vi "HMI-Reactor.vi"() -> ()   [LabVIEW 2018]
uses:
  <vilib>/Platform/TimedLoop/XDataNode/timing_clust.ctl
  <vilib>/Platform/TimedLoop/XDataNode/nitl_modes.ctl
  <vilib>/Platform/TimedLoop/XDataNode/wakeup.ctl
  <vilib>/Modbus/master/Create Master Instance (TCP).vi
  <vilib>/Modbus/master/Modbus Master.lvclass
  <vilib>/Platform/TimedLoop/XDataNode/XDataNode.xnode
  <vilib>/Platform/TimedLoop/XDataNode/XDNodeRunTimeDep.lvlib
panel:
  out "BPCS-10HIC100":dbl
  out "BPCS-10TIC100-SP":dbl
  out "BPCS-10TIC100-KD":dbl
  out "BPCS-10TIC100-KI":dbl
  out "BPCS-10TIC100-KP":dbl
  out "BPCS-10HIC200":dbl
  out "BPCS-10LIC200-SP":dbl
  out "BPCS-10LIC200-KD":dbl
  out "BPCS-10LIC200-KI":dbl
  out "BPCS-10LIC200-KP":dbl
  out "BPCS-10HIC300":dbl
  in  "cast type 3":dbl[](array[numeric])
  out "M2":bool
  out "M1":bool
  in  "type":u16[](array[numeric])
  in  "cast type 2":dbl[](array[numeric])
  out "F":dbl
  in  "cast type":dbl[](array[numeric])
  out "CA":dbl=456.3558684423593 format="%#_3g"
  out "CA0":dbl=2000.0 format="%#_3g"
  out "10SDV502":bool=TRUE
  out "?":dbl format="%#_3g"
  in  "10HIC300":dbl=50.0
  out "TJ":dbl=365.3749789937039 format="%#_3g"
  out "T":dbl=333.97788169438996 format="%#_3g"
  out "Reactor Temp":T1={"% Opening"=0.0, "SP"=0.0, "Reactor Temp"=333.97788169438996, "Temp"=333.97788169438996} {"Temp" format="%#_4g"; "Reactor Temp" scale=0.0..700.0; "SP" scale=0.0..700.0; "% Opening" scale=0.0..100.0}
  in  "10TIC100 Faceplate":T2={"PID Parameters"={"KP"=-1.0, "KI"=0.5, "KD"=0.0}, "M"=FALSE, "SP_VAL"=0.0, "% Open"=50.0}
  out "?":dbl format="%#_3g"
  out "10SDV501":bool=TRUE
  out "FJ":dbl=15.0 format="%#_3g"
  out "TJ0":dbl=300.0 format="%#_3g"
  out "10SDV500":bool=TRUE
  out "F0":dbl=1.0 format="%#_3g"
  out "T0":dbl=323.0 format="%#_3g"
  out "Reactor Level":T3={"% Opening"=0.0, "SP"=0.0, "Reactor Level"=54.508701366151044, "Level"=54.508701366151044} {"Level" format="%#_4g"; "Reactor Level" scale=0.0..100.0; "SP" scale=0.0..100.0; "% Opening" scale=0.0..100.0}
  out "?":dbl format="%#_3g"
  in  "10LIC200 Faceplate":T2={"PID Parameters"={"KP"=8.0, "KI"=0.4, "KD"=0.0}, "M"=FALSE, "SP_VAL"=0.0, "% Open"=50.0}
  out "10-R-100":dbl(slide)=54.508701366151044 scale=0.0..100.0 scale format="%#_4g"
  in  "stop":bool
  # "LIC = level controller"
  # "feed flow"
  # "Reactant inlet concentration"
  # "m3/min"
  # "10LV200"
  # "Mole/m3"
  # "%"
  # "K"
  # "%"
  # "K"
  # "TIC=Temperature controller"
  # "coolant flow"
  # "m3/min"
  # "10TV100"
  # "%"
  # "K"
  # "Mole/m3"
  # "%"
  # "K"
  # "coolant inlet temp"
  # "A"
  # "%"
  # "A"
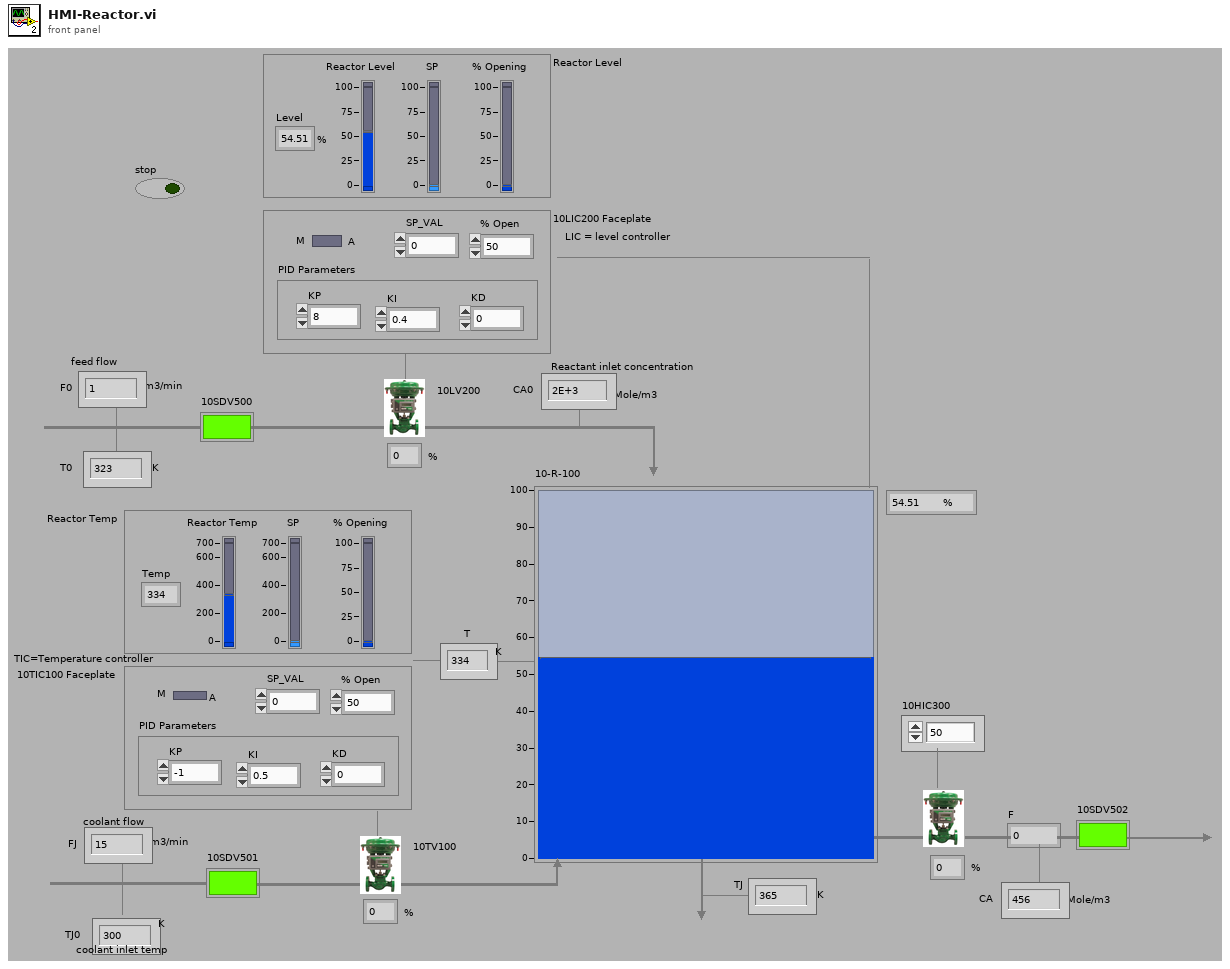
[diagram p1: front panel]
types:
  T1 = cluster{"% Opening":dbl, "SP":dbl, "Reactor Temp":dbl, "Temp":dbl}
  T2 = cluster{"PID Parameters":cluster{"KP":dbl, "KI":dbl, "KD":dbl}, "M":bool, "SP_VAL":dbl, "% Open":dbl}
  T3 = cluster{"% Opening":dbl, "SP":dbl, "Reactor Level":dbl, "Level":dbl}
  T4 = typedef "XDNodeRunTimeDep.lvlib/timing_clust.ctl" = cluster{"Expected End [f-1]":u64, "Actual End [f-1]":u64, "Finished Late? [f-1]":bool, "Expected End [i-1]":u64, "Actual End [i-1]":u64, "Finished Late? [i-1]":bool, "Expected Start [i]":u64, "Actual Start [i]":u64, "Expected Start [f]":u64, "Actual Start [f]":u64, "Source Name":string, "Structure Name":string, "Period":i64, "Deadline":i64, "Offset":i64, "Start":i64, "Priority":i32, "Timeout":i32, "Mode":T5, "Wakeup Reason":T6, "Error":errorcluster, "Source Type":string, "Secondary Source Type":string, "Global End Time":u64, "Global Start Time":u64, "Frame Duration":u64, "Iteration Duration":u64, "Assigned CPU":i32, "I/O Scan Engine Mode":u32}
  T5 = typedef "XDNodeRunTimeDep.lvlib/nitl_modes.ctl" = enum32{"No Change", "Process missed periods, maintain original phase", "Discard missed periods, maintain original phase", "Process missed periods, ignore original phase", "Discard missed periods, ignore original phase"}
  T6 = typedef "XDNodeRunTimeDep.lvlib/wakeup.ctl" = enum32{"Normal", "Aborted", "Asynchronous wakeup", "Timing source error", "Timed loop error", "Timeout"}
  T7 = cluster{"% Open":dbl, "SP_VAL":dbl, "Numeric":dbl, "Numeric":dbl}
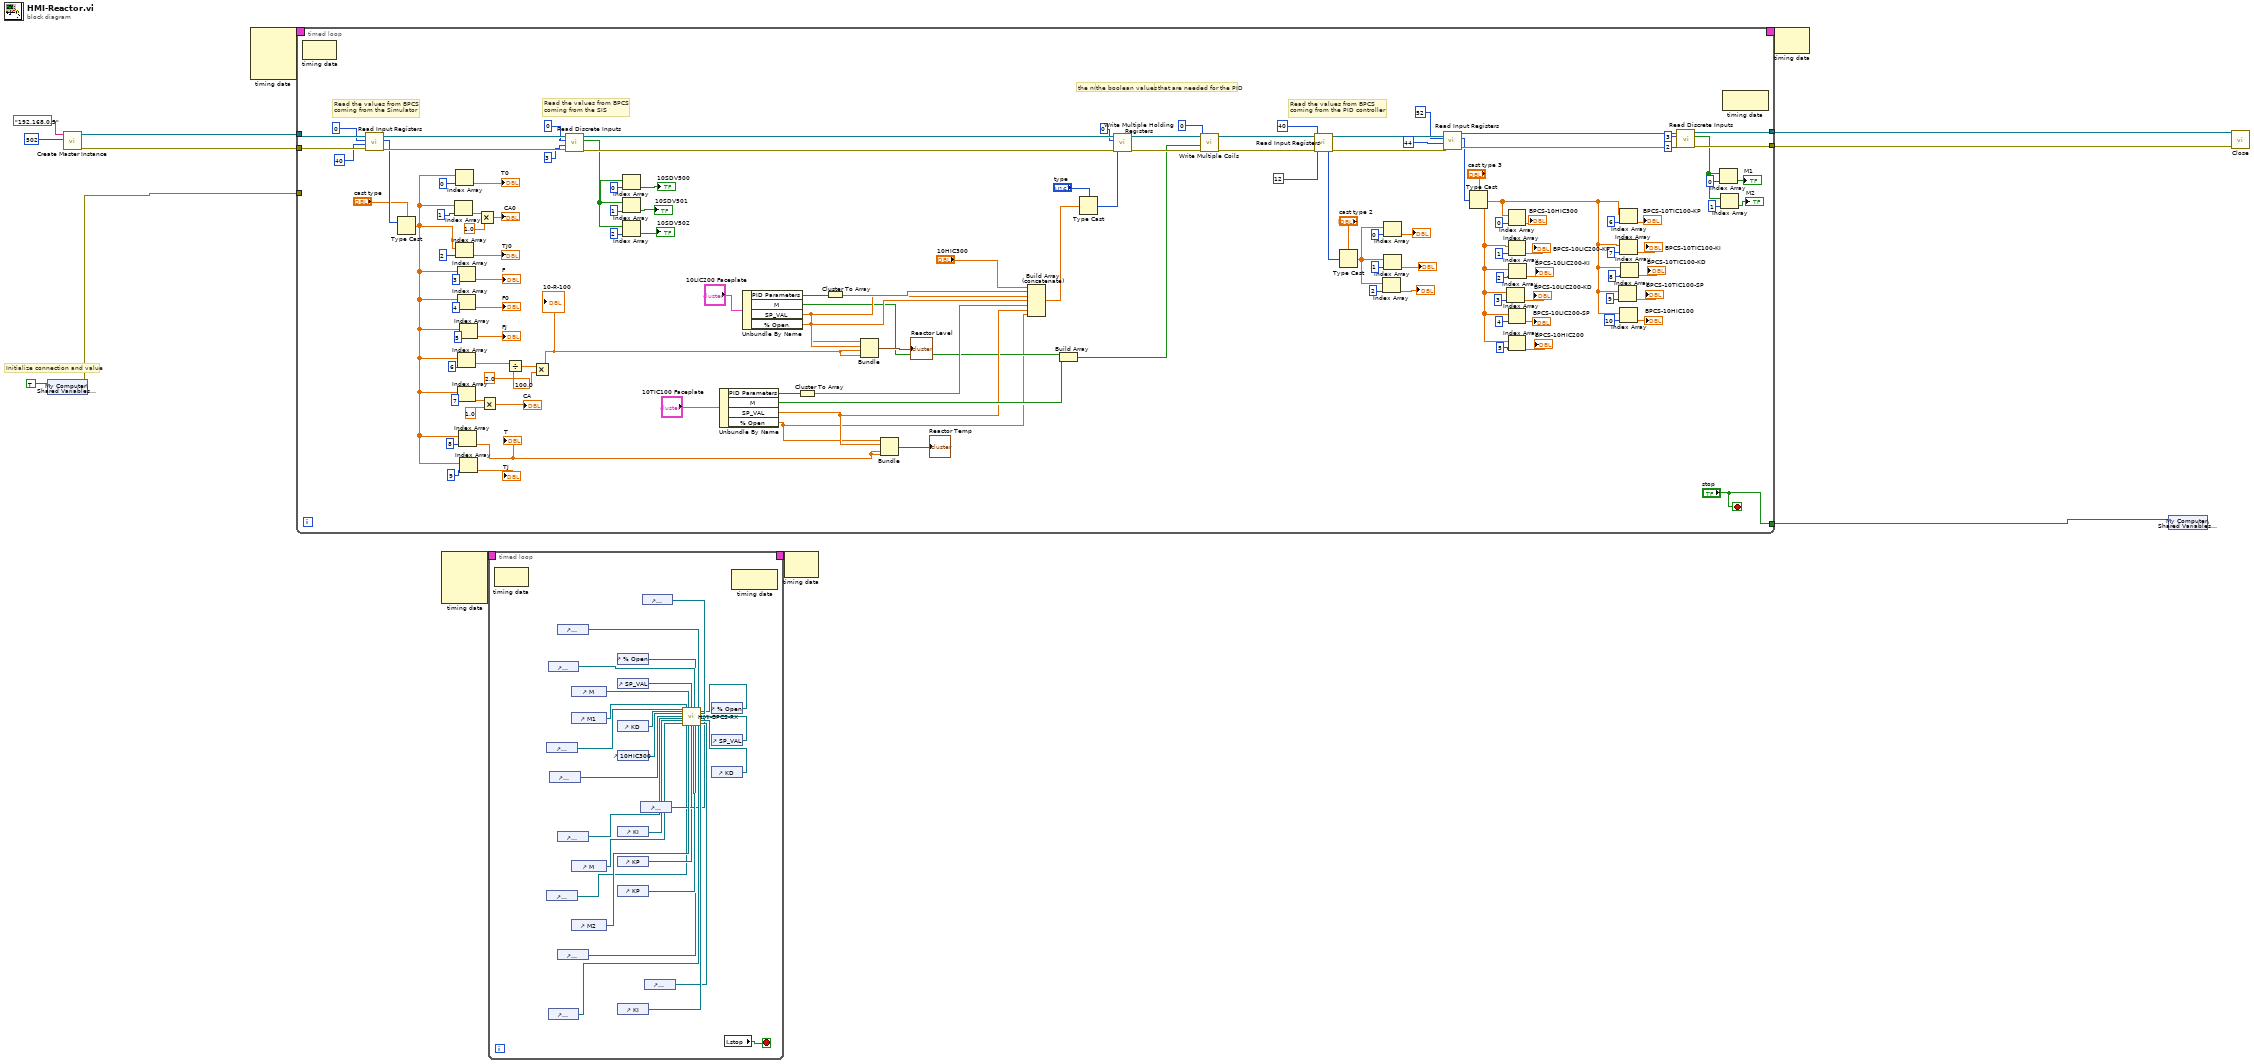
[diagram p0: block diagram]
diagram:
  # "Initialize connection and value"
  n1 = shared-variable "My Computer\\Shared Variables.lvlib\\stop"(TRUE) -> (error out=w12:errorcluster)  [unwired: 1 in]
  n2 = call-poly <vilib>:"Create Master Instance.vi"("port (502)"=u16 502, "address"="192.168.0.5") -> ("error out"=w7:errorcluster, "TCP master instance"=w8:refnum<class "Modbus Master.lvclass">)  [unwired: 8 in]
  n3 = node-c288() -> (w6:T4)  [unwired: 4 in]
  n4 = timed-loop {
    tunnel: ["stop"] -> w13
    tunnel: w12 -> [_]
    tunnel: w8 -> [w138]
    tunnel: w7 -> [w137]
    timing: w6 -> [_]
    timing-out: [_] -> w5
    tunnel: [w136] -> w4
    tunnel: [w135] -> w3
    stop <- "stop" stop-if-true
    # "Read the values from BPCS \ncoming from the PID controller"
    # "the boolean values"
    # "the numeric values"
    # "send the values to BPCS  that are needed for the PID"
    # "Read the values from BPCS \ncoming from the SIS"
    # "Read the values from BPCS \ncoming from the Simulator"
    n5 = node-c288() -> ()  [unwired: 1 in, 1 out]
    n6 = call-dynamic "Read Input Registers.vi"("error in (no error)"=w137, "number of input registers"=u16 40, "starting address"=u16 0, "Modbus master in"=w138) -> ("error out"=w132:errorcluster, "register values"=w121:u16[], "Modbus master out"=w133:refnum<class "Modbus Master.lvclass">)  [unwired: 5 in]
    n7 = Type Cast(type="cast type", x=w121) -> (*(type *) &x=w98:dbl[])
    n8 = Index Array(array=w98, index=1) -> (element=w117:dbl)
    n9 = Index Array "Index Array"(array=w98, index=0) -> (element=→"T0":dbl)
    n10 = Index Array(array=w98, index=2) -> (element=→"TJ0":dbl)
    n11 = Index Array(array=w98, index=3) -> (element=→"F":dbl)
    n12 = Index Array(array=w98, index=6) -> (element=w100:dbl)
    n13 = Index Array(array=w98, index=4) -> (element=→"F0":dbl)
    n14 = Index Array(array=w98, index=7) -> (element=w101:dbl)
    n15 = Index Array(array=w98, index=8) -> (element=w14:dbl)
    "T" <- w14
    n16 = Index Array(array=w98, index=5) -> (element=→"FJ":dbl)
    n17 = Index Array(array=w98, index=9) -> (element=→"TJ":dbl)
    n18 = Multiply(x=w117, y=1.0) -> (x*y=→"CA0":dbl)
    n19 = Multiply(x=w101, y=1.0) -> (x*y=→"CA":dbl)
    n20 = Divide(x=w100, y=2.0 ("x")) -> (x/y=w125:dbl)
    n21 = Multiply(x=w125, y=100.0) -> (x*y=w129:dbl)
    "10-R-100" <- w129
    n22 = call-dynamic "Read Discrete Inputs.vi"("error in (no error)"=w132, "number of discrete inputs"=u16 3, "starting address"=u16 0, "Modbus master in"=w133) -> ("error out"=w130:errorcluster, "discrete input values"=w96:bool[], "Modbus master out"=w131:refnum<class "Modbus Master.lvclass">)  [unwired: 5 in]
    n23 = Index Array(array=w96, index=0) -> (element=→"10SDV500":bool)
    n24 = Index Array(array=w96, index=1) -> (element=→"10SDV501":bool)
    n25 = Index Array(array=w96, index=2) -> (element=→"10SDV502":bool)
    n26 = Unbundle By Name("10TIC100 Faceplate") -> ("PID Parameters"=w81:cluster{"KP":dbl, "KI":dbl, "KD":dbl}, "M"=w85:bool, "SP_VAL"=w73:dbl, "% Open"=w15:dbl)
    n27 = Unbundle By Name("10LIC200 Faceplate") -> ("PID Parameters"=w83:cluster{"KP":dbl, "KI":dbl, "KD":dbl}, "M"=w49:bool, "SP_VAL"=w76:dbl, "% Open"=w75:dbl)
    n28 = Cluster To Array(cluster=w81) -> (array=w74:dbl[])
    n29 = Cluster To Array(cluster=w83) -> (array=w77:dbl[])
    n30 = Bundle("% Open"=w75, "SP_VAL"=w76, w129, w129) -> (→"Reactor Level":cluster{"% Open":dbl, "SP_VAL":dbl, dbl, dbl})  [unwired: 1 in]
    n31 = Bundle("% Open"=w15, "SP_VAL"=w73, "Numeric"=w14, "Numeric"=w14) -> (→"Reactor Temp":T7)  [unwired: 1 in]
    n32 = Build Array (concatenate)("10HIC300", w77, w76, w75, w74, w73, w15) -> (w72:dbl[])
    n33 = Build Array(w49, w85) -> (w69:bool[])
    n34 = Type Cast(type="type", x=w72) -> (*(type *) &x=w79:u16[])
    n35 = call-dynamic "Write Multiple Holding Registers.vi"("error in (no error)"=w130, "holding register values"=w79, "starting address"=u16 0, "Modbus master in"=w131) -> ("error out"=w70:errorcluster, "Modbus master out"=w71:refnum<class "Modbus Master.lvclass">)  [unwired: 6 in]
    n36 = call-dynamic "Write Multiple Coils.vi"("error in (no error)"=w70, "coil values"=w69, "starting address"=u16 0, "Modbus master in"=w71) -> ("error out"=w127:errorcluster, "Modbus master out"=w128:refnum<class "Modbus Master.lvclass">)  [unwired: 6 in]
    n37 = call-dynamic "Read Input Registers.vi"("error in (no error)"=w127, "number of input registers"=u16 12, "starting address"=u16 40, "Modbus master in"=w128) -> ("error out"=w46:errorcluster, "register values"=w59:u16[], "Modbus master out"=w47:refnum<class "Modbus Master.lvclass">)  [unwired: 5 in]
    n38 = Type Cast(type="cast type 2", x=w59) -> (*(type *) &x=w50:dbl[])
    n39 = Index Array(array=w50, index=2) -> (element=→"?":dbl)
    n40 = Index Array(array=w50, index=0) -> (element=→"?":dbl)
    n41 = Index Array "Index Array"(array=w50, index=1) -> (element=→"?":dbl)
    n42 = call-dynamic "Read Input Registers.vi"("error in (no error)"=w46, "number of input registers"=u16 44, "starting address"=u16 52, "Modbus master in"=w47) -> ("error out"=w44:errorcluster, "register values"=w34:u16[], "Modbus master out"=w45:refnum<class "Modbus Master.lvclass">)  [unwired: 5 in]
    n43 = Type Cast(type="cast type 3", x=w34) -> (*(type *) &x=w28:dbl[])
    n44 = Index Array(array=w28, index=3) -> (element=→"BPCS-10LIC200-KD":dbl)
    n45 = Index Array(array=w28, index=0) -> (element=→"BPCS-10HIC300":dbl)
    n46 = Index Array(array=w28, index=1) -> (element=→"BPCS-10LIC200-KP":dbl)
    n47 = Index Array(array=w28, index=4) -> (element=→"BPCS-10LIC200-SP":dbl)
    n48 = Index Array(array=w28, index=5) -> (element=→"BPCS-10HIC200":dbl)
    n49 = Index Array(array=w28, index=2) -> (element=→"BPCS-10LIC200-KI":dbl)
    n50 = Index Array(array=w28, index=9) -> (element=→"BPCS-10TIC100-SP":dbl)
    n51 = Index Array(array=w28, index=6) -> (element=→"BPCS-10TIC100-KP":dbl)
    n52 = Index Array(array=w28, index=7) -> (element=→"BPCS-10TIC100-KI":dbl)
    n53 = Index Array(array=w28, index=10) -> (element=→"BPCS-10HIC100":dbl)
    n54 = Index Array(array=w28, index=8) -> (element=→"BPCS-10TIC100-KD":dbl)
    n55 = call-dynamic "Read Discrete Inputs.vi"("error in (no error)"=w44, "number of discrete inputs"=u16 2, "starting address"=u16 3, "Modbus master in"=w45) -> ("error out"=w135:errorcluster, "discrete input values"=w63:bool[], "Modbus master out"=w136:refnum<class "Modbus Master.lvclass">)  [unwired: 5 in]
    n56 = Index Array(array=w63, index=0) -> (element=→"M1":bool)
    n57 = Index Array(array=w63, index=1) -> (element=→"M2":bool)
    n58 = node-c288() -> ()  [unwired: 1 in, 1 out]
  }
  n59 = node-c288() -> (w2:T4)  [unwired: 4 in]
  n60 = timed-loop {
    timing: w2 -> [_]
    timing-out: [_] -> w1
    stop <- w167 stop-if-true
    n61 = node-c288() -> ()  [unwired: 1 in, 1 out]
    n62 = control-ref of="BPCS-10TIC100-KD"() -> (w145:refnum<vi>)
    n63 = control-ref of="BPCS-10TIC100-KP"() -> (w149:refnum<vi>)
    n64 = control-ref of="BPCS-10TIC100-SP"() -> (w143:refnum<vi>)
    n65 = control-ref of="BPCS-10LIC200-KP"() -> (w159:refnum<vi>)
    n66 = control-ref of="BPCS-10TIC100-KI"() -> (w147:refnum<vi>)
    n67 = control-ref of="BPCS-10HIC100"() -> (w141:refnum<vi>)
    n68 = control-ref of="BPCS-10HIC300"() -> (w163:refnum<vi>)
    n69 = control-ref of="BPCS-10HIC200"() -> (w151:refnum<vi>)
    n70 = control-ref of="M"() -> (w166:refnum<vi>)
    n71 = control-ref of="M1"() -> (w165:refnum<vi>)
    n72 = control-ref of="M"() -> (w162:refnum<vi>)
    n73 = control-ref of="M2"() -> (w161:refnum<vi>)
    n74 = control-ref of="% Open"() -> (w142:refnum<vi>)
    n75 = control-ref of="SP_VAL"() -> (w144:refnum<vi>)
    n76 = control-ref of="KD"() -> (w146:refnum<vi>)
    n77 = control-ref of="10HIC300"() -> (w164:refnum<vi>)
    n78 = control-ref of="KI"() -> (w148:refnum<vi>)
    n79 = control-ref of="KP"() -> (w150:refnum<vi>)
    n80 = control-ref of="KP"() -> (w160:refnum<vi>)
    n81 = control-ref of="KI"() -> (w158:refnum<vi>)
    n82 = control-ref of="BPCS-10LIC200-KD"() -> (w155:refnum<vi>)
    n83 = control-ref of="BPCS-10LIC200-SP"() -> (w153:refnum<vi>)
    n84 = control-ref of="BPCS-10LIC200-KI"() -> (w157:refnum<vi>)
    n85 = control-ref of="% Open"() -> (w152:refnum<vi>)
    n86 = control-ref of="SP_VAL"() -> (w154:refnum<vi>)
    n87 = control-ref of="KD"() -> (w156:refnum<vi>)
    n88 = call "HMI-BPCS-RX.vi"("Digital in"=w145, "DigNum Refnum 9"=w146, "DigNum Refnum"=w164, "reference 10"=w147, "reference 2"=w163, "DigNum Refnum 8"=w148, "Bool Refnum 2"=w162, "reference"=w165, "reference 9"=w149, "Bool Refnum"=w166, "reference 3"=w161, "DigNum Refnum 10"=w144, "DigNum Refnum 7"=w150, "reference 12"=w143, "DigNum Refnum 2"=w160, "DigNum Refnum 11"=w142, "reference 8"=w151, "reference 13"=w141, "reference 4"=w159, "DigNum Refnum 6"=w152, "reference 7"=w153, "DigNum Refnum 5"=w154, "reference 6"=w155, "DigNum Refnum 4"=w156, "reference 5"=w157, "DigNum Refnum 3"=w158) -> ()  [unwired: 2 in]
    n89 = local read "stop"() -> (w167:bool)
    n90 = node-c288() -> ()  [unwired: 1 in, 1 out]
  }
  n91 = node-c288(w1) -> ()  [unwired: 1 out]
  n92 = node-c288(w5) -> ()  [unwired: 1 out]
  n93 = shared-variable "My Computer\\Shared Variables.lvlib\\stop"(w13) -> ()  [unwired: 1 in, 1 out]
  n94 = call-dynamic "Close.vi"("error in (no error)"=w3, "Modbus master in"=w4) -> ()  [unwired: 9 in, 1 out]
